vi "Progess bar.vi"(5 "Time out (s)":i32=15, 7 "error in":errorcluster, 9 "Duration (s)":u32=5) -> (0 "error out":errorcluster)   [LabVIEW 2021]
uses:
  Progress bar.ctl
  <vilib>/NI/Progress Bar/Controls/Progress Bar Properties.ctl
  <vilib>/NI/Progress Bar/Controls/Update Bar Actions.ctl
  7d7f576e-4f50-4eb2-9903-a620b73bda78.vi
  Support Globals.vi
  <vilib>/NI/Progress Bar/Progress Bar.lvlib
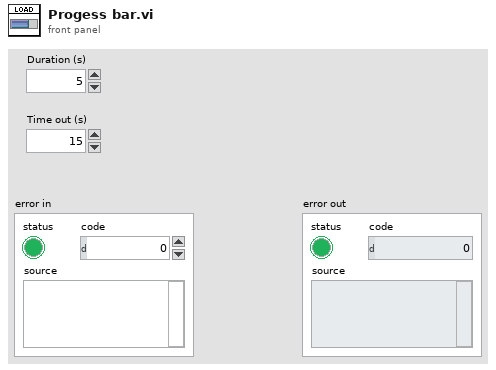
[diagram p1: front panel]
types:
  T1 = typedef "Progress bar.ctl" = enum16{"Init", "Auto", "Set", "Add", "Delay", "Close"}
  T2 = typedef "Progress Bar.lvlib/Update Bar Actions.ctl" = enum16{"Add To Existing", "Set to Value"}
  T3 = typedef "Progress Bar.lvlib/Progress Bar Properties.ctl" = cluster{"Background Color":u32, "Installer Title":string, "Title Color":u32, "Action Text":string, "Text Color":u32, "Slider Value":u8, "Bar Color":u32, "Timeout":i32}
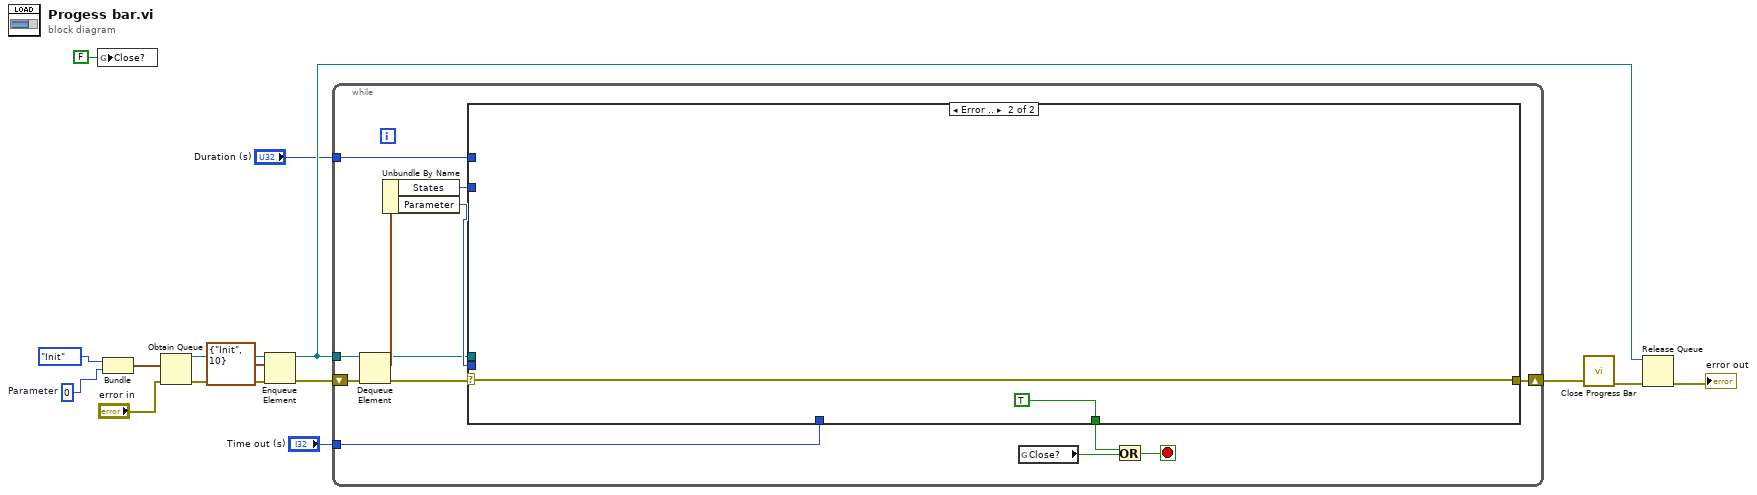
[diagram p0: block diagram]
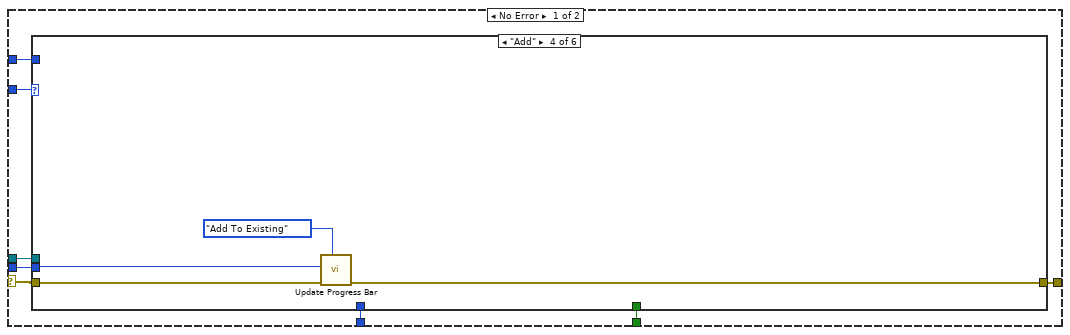
[diagram p2: hidden frame]
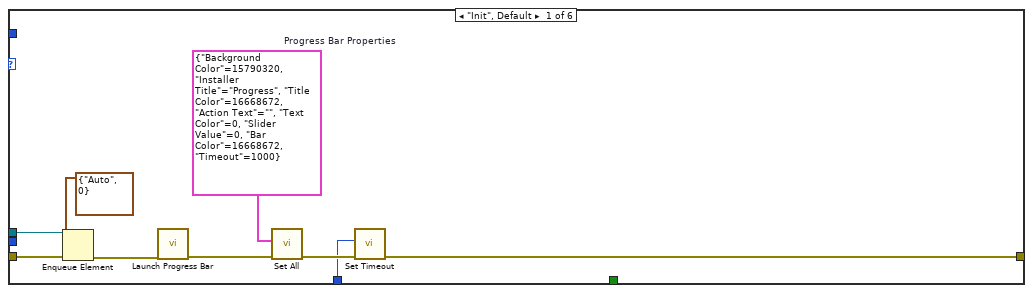
[diagram p3: hidden frame]
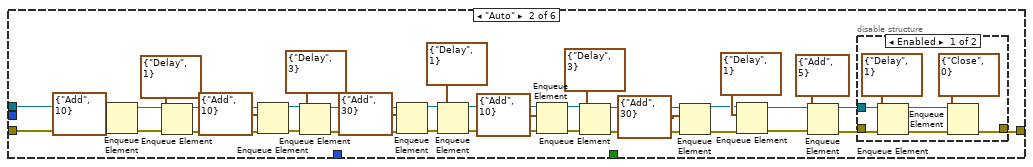
[diagram p4: hidden frame]
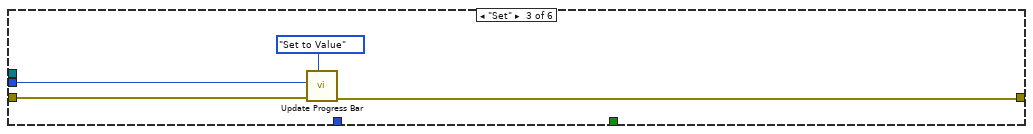
[diagram p6: hidden frame]
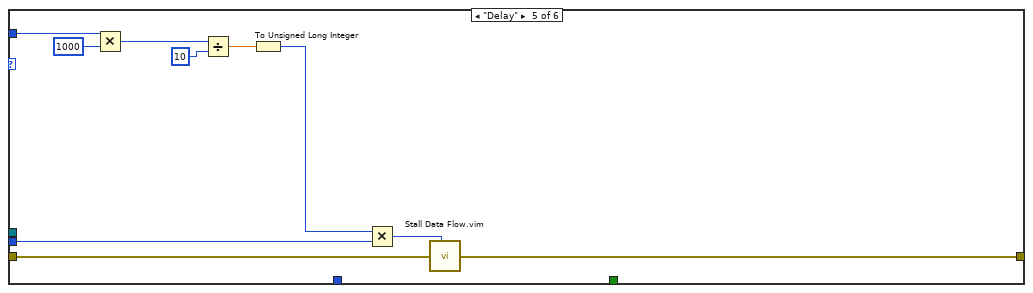
[diagram p7: hidden frame]
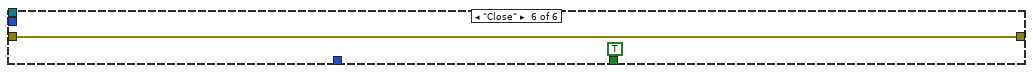
[diagram p8: hidden frame]
diagram:
  w13 = 0  # Parameter
  n1 = global write "Support Globals.vi" "Close?"(FALSE ("Close?")) -> ()
  n2 = Bundle("States"=Progress_bar."Init", "Parameter"=w13) -> (w15:cluster{"States":T1, "Parameter":i32})  [unwired: 1 in]
  n3 = Obtain Queue(element data type=w15, error in (no error)="error in") -> (queue out=w12:refnum<queue>, error out=w9:errorcluster)  [unwired: 3 in, 1 out]
  n4 = Enqueue Element(queue=w12, element=cluster{"States":T1, i32} {"States"=enum."Init", 10}, error in (no error)=w9) -> (queue out=w6:refnum<queue>, error out=w8:errorcluster)  [unwired: 1 in, 1 out]
  n5 = while {
    shift-right: [w28] -> w3
    shift-left: w8 -> [w27]
    tunnel: w6 -> [w25]
    tunnel: "Time out (s)" -> [w23]
    tunnel: "Duration (s)" -> [w16]
    stop <- w21 stop-if-true
    n6 = Dequeue Element(queue=w25, error in (no error)=w27) -> (queue out=w17:refnum<queue>, element=w22:cluster{"States":T1, "Parameter":i32}, error out=w26:errorcluster)  [unwired: 1 in, 1 out]
    n7 = Unbundle By Name(w22) -> ("States"=w24:T1, "Parameter"=w18:i32)
    n8 = case shown="Error .." w26 {
      selector: w26 -> [w35 w110]
      tunnel: [w36 w110] -> w28
      tunnel: w24 -> [w34 _]
      tunnel: w23 -> [w33 _]
      tunnel: [w32 TRUE] -> w20
      tunnel: w18 -> [w31 _]
      tunnel: w17 -> [w30 _]
      tunnel: w16 -> [w29 _]
      frame No Error {
        n9 = case shown="\"Add\"" w34 {
          tunnel: w35 -> [w39 w56 w92 w97 w107 w108]
          tunnel: [w43 w75 w93 w96 w106 w108] -> w36
          tunnel: w33 -> [w41 _ _ _ _ _]
          tunnel: [_ _ _ _ _ TRUE] -> w32
          tunnel: w31 -> [_ _ w90 w95 w102 _]
          tunnel: w30 -> [w40 w81 _ _ _ _]
          tunnel: w29 -> [_ _ _ _ w100 _]
          frame "Init", Default {
            w42 = T3 {"Background Color"=15790320, "Installer Title"="Progress", "Title Color"=16668672, "Action Text"="", "Text Color"=0, "Slider Value"=0, "Bar Color"=16668672, "Timeout"=1000}  # Progress Bar Properties
            n10 = Enqueue Element(queue=w40, element=cluster{"States":T1, "Parameter":i32} {"States"=enum."Auto", "Parameter"=0}, error in (no error)=w39) -> (error out=w38:errorcluster)  [unwired: 1 in, 2 out]
            n11 = call <vilib>:"Launch Progress Bar.vi"("error in (no error)"=w38) -> ("error out"=w45:errorcluster)  [unwired: 9 in, 1 out]
            n12 = call <vilib>:"Set All.vi"("error in (no error)"=w45, "Progress Bar Properties (Default)"=w42) -> ("error out"=w44:errorcluster)  [unwired: 9 in]
            n13 = call <vilib>:"Set Timeout.vi"("error in (no error)"=w44, "Timeout"=w41) -> ("error out"=w43:errorcluster)  [unwired: 9 in]
          }
          frame "Auto" {
            n14 = Enqueue Element(queue=w81, element=cluster{"States":T1, "Parameter":i32} {"States"=enum."Add", "Parameter"=10}, error in (no error)=w56) -> (queue out=w59:refnum<queue>, error out=w60:errorcluster)  [unwired: 1 in, 1 out]
            n15 = Enqueue Element(queue=w59, element=cluster{"States":T1, "Parameter":i32} {"States"=enum."Delay", "Parameter"=1}, error in (no error)=w60) -> (queue out=w58:refnum<queue>, error out=w55:errorcluster)  [unwired: 1 in, 1 out]
            n16 = Enqueue Element(queue=w58, element=cluster{"States":T1, "Parameter":i32} {"States"=enum."Add", "Parameter"=10}, error in (no error)=w55) -> (queue out=w63:refnum<queue>, error out=w54:errorcluster)  [unwired: 1 in, 1 out]
            n17 = Enqueue Element(queue=w63, element=cluster{"States":T1, "Parameter":i32} {"States"=enum."Delay", "Parameter"=3}, error in (no error)=w54) -> (queue out=w62:refnum<queue>, error out=w53:errorcluster)  [unwired: 1 in, 1 out]
            n18 = Enqueue Element(queue=w62, element=cluster{"States":T1, "Parameter":i32} {"States"=enum."Add", "Parameter"=30}, error in (no error)=w53) -> (queue out=w66:refnum<queue>, error out=w52:errorcluster)  [unwired: 1 in, 1 out]
            n19 = Enqueue Element(queue=w66, element=cluster{"States":T1, "Parameter":i32} {"States"=enum."Delay", "Parameter"=1}, error in (no error)=w52) -> (queue out=w65:refnum<queue>, error out=w51:errorcluster)  [unwired: 1 in, 1 out]
            n20 = Enqueue Element(queue=w65, element=cluster{"States":T1, "Parameter":i32} {"States"=enum."Add", "Parameter"=10}, error in (no error)=w51) -> (queue out=w69:refnum<queue>, error out=w50:errorcluster)  [unwired: 1 in, 1 out]
            n21 = Enqueue Element(queue=w69, element=cluster{"States":T1, "Parameter":i32} {"States"=enum."Delay", "Parameter"=3}, error in (no error)=w50) -> (queue out=w68:refnum<queue>, error out=w49:errorcluster)  [unwired: 1 in, 1 out]
            n22 = Enqueue Element(queue=w68, element=cluster{"States":T1, "Parameter":i32} {"States"=enum."Add", "Parameter"=30}, error in (no error)=w49) -> (queue out=w70:refnum<queue>, error out=w71:errorcluster)  [unwired: 1 in, 1 out]
            n23 = Enqueue Element(queue=w70, element=cluster{"States":T1, "Parameter":i32} {"States"=enum."Delay", "Parameter"=1}, error in (no error)=w71) -> (queue out=w73:refnum<queue>, error out=w48:errorcluster)  [unwired: 1 in, 1 out]
            n24 = Enqueue Element(queue=w73, element=cluster{"States":T1, "Parameter":i32} {"States"=enum."Add", "Parameter"=5}, error in (no error)=w48) -> (queue out=w74:refnum<queue>, error out=w47:errorcluster)  [unwired: 1 in, 1 out]
            n25 = disable-structure shown="Enabled" {
              disable-tunnel: [w88 w89] -> w75
              disable-tunnel: w74 -> [w86 _]
              disable-tunnel: w47 -> [w83 w89]
              frame Enabled {
                n26 = Enqueue Element(queue=w86, element=cluster{"States":T1, "Parameter":i32} {"States"=enum."Delay", "Parameter"=1}, error in (no error)=w83) -> (queue out=w87:refnum<queue>, error out=w82:errorcluster)  [unwired: 1 in, 1 out]
                n27 = Enqueue Element(queue=w87, element=cluster{"States":T1, "Parameter":i32} {"States"=enum."Close", "Parameter"=0}, error in (no error)=w82) -> (error out=w88:errorcluster)  [unwired: 1 in, 2 out]
              }
              frame Disabled {
              }
            }
          }
          frame "Set" {
            n28 = call <vilib>:"Update Progress Bar.vi"("Action"=Update_Bar_Actions."Set to Value", "error in (no error)"=w92, "Value"=w90) -> ("error out"=w93:errorcluster)  [unwired: 8 in]
          }
          frame "Add" {
            n29 = call <vilib>:"Update Progress Bar.vi"("Action"=Update_Bar_Actions."Add To Existing", "error in (no error)"=w97, "Value"=w95) -> ("error out"=w96:errorcluster)  [unwired: 8 in]
          }
          frame "Delay" {
            n30 = Multiply(x=w100, y=u32 1000) -> (x*y=w98:u32)
            n31 = Divide(x=w98, y=10) -> (x/y=w105:dbl)
            n32 = To Unsigned Long Integer(number=w105) -> (unsigned 32bit integer=w103:u32)
            n33 = Multiply(x=w103, y=w102) -> (x*y=w101:u32)
            n34 = call "Stall Data Flow.vim"("value in"=w107, "milliseconds to wait"=w101) -> ("value out"=w106:errorcluster)  [unwired: 1 out]
          }
          frame "Close" {
          }
        }
      }
      frame Error {
      }
    }
    n35 = global read "Support Globals.vi" "Close?"() -> (w19:bool)
    n36 = Or(x=w20, y=w19) -> (x .or. y?=w21:bool)
  }
  n37 = call <vilib>:"Close Progress Bar.vi"("error in (no error)"=w3) -> ("error out"=w2:errorcluster)  [unwired: 9 in, 1 out]
  n38 = Release Queue(queue=w6, error in (no error)=w2) -> (error out=→"error out":errorcluster)  [unwired: 1 in, 2 out]
